vi "MTMount_putSample_DynaleneCooling.vi"(8 "error in (no error)":errorcluster, 11 "Dynalene_Cooling_Ctl":T1) -> (0 "error out":errorcluster, 2 "function return":i32, 3 "Dynalene_Cooling_Ctl out":T1)   [LabVIEW 2018, in "SALLV_MTMount.lvlib"]
doc: "int MTMount_shm_putSample_Dynalene_CoolingLV(MTMount_Dynalene_CoolingLV *Dynalene_Cooling_Ctl );"
uses:
  SALLV_MTMount.lvlib
  DataTypes/Dynalene_Cooling.ctl
  SALLV_MTMount.so
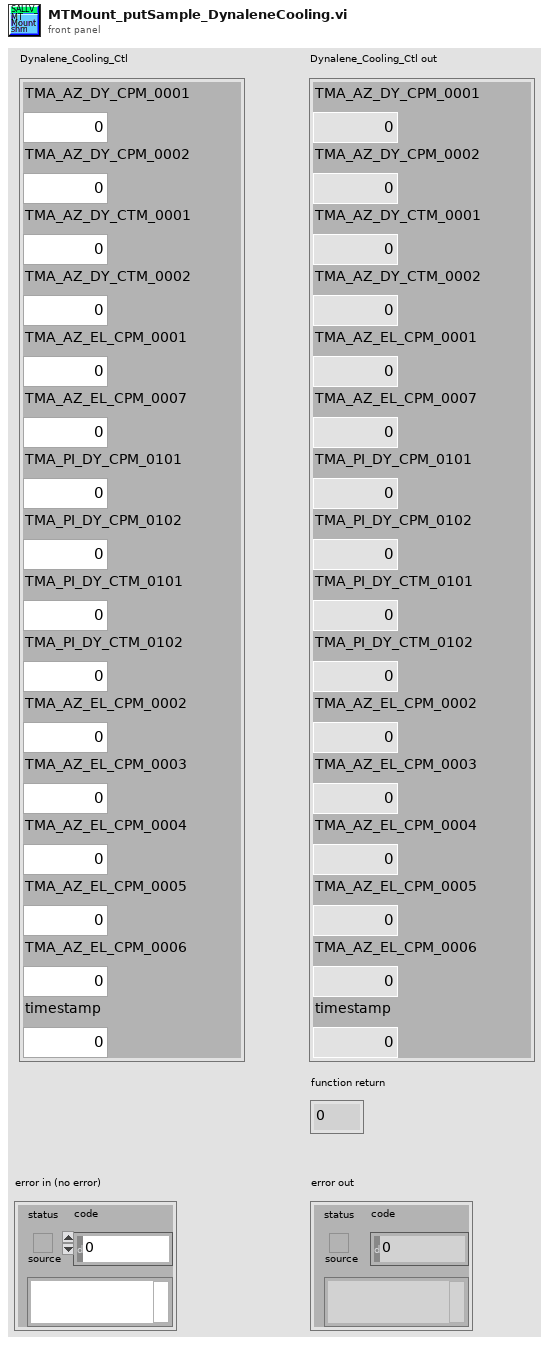
[diagram p1: front panel]
types:
  T1 = typedef "SALLV_MTMount.lvlib/Dynalene_Cooling.ctl" = cluster{"TMA_AZ_DY_CPM_0001":dbl, "TMA_AZ_DY_CPM_0002":dbl, "TMA_AZ_DY_CTM_0001":dbl, "TMA_AZ_DY_CTM_0002":dbl, "TMA_AZ_EL_CPM_0001":dbl, "TMA_AZ_EL_CPM_0007":dbl, "TMA_PI_DY_CPM_0101":dbl, "TMA_PI_DY_CPM_0102":dbl, "TMA_PI_DY_CTM_0101":dbl, "TMA_PI_DY_CTM_0102":dbl, "TMA_AZ_EL_CPM_0002":dbl, "TMA_AZ_EL_CPM_0003":dbl, "TMA_AZ_EL_CPM_0004":dbl, "TMA_AZ_EL_CPM_0005":dbl, "TMA_AZ_EL_CPM_0006":dbl, "timestamp":dbl}
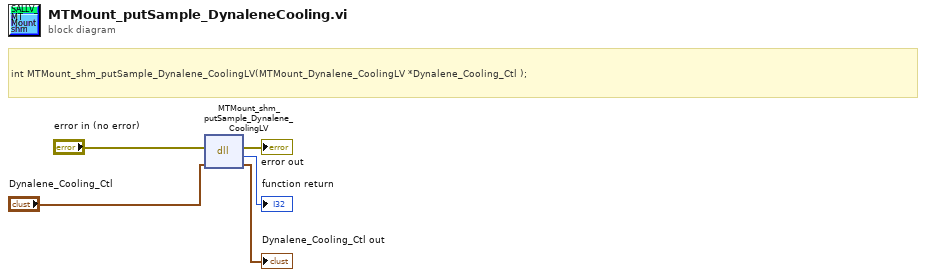
[diagram p0: block diagram]
diagram:
  # "int MTMount_shm_putSample_Dynalene_CoolingLV(MTMount_Dynalene_CoolingLV *Dynalene_Cooling_Ctl );"
  n1 = dll-call lib="home/ttsai/Document/salApiMTMount/SALLV_MTMount/SALLV_MTMount.*" fn="MTMount_shm_putSample_Dynalene_CoolingLV"(error in="error in (no error)", "Dynalene_Cooling_Ctl"="Dynalene_Cooling_Ctl") -> (error out=→"error out":errorcluster, →"function return":i32, "Dynalene_Cooling_Ctl"=→"Dynalene_Cooling_Ctl out":T1)  [unwired: 2 in, 1 out]
